vi "op-selector.vi"(6 "Channel":T1={"Operation"=0, "Num. Steps"=0, "Begin"=0.0, "Step Size"=0.0, "Input - A"=0, "Input - B"=0, "Output - LO"=0.0, "Output - HI"=0.0, "Reset"=FALSE, "Analog Output"=0, "Trigger Input"=0, "Initialize To"=0, "Digital Inputs"=[0, 0, 0, 0, 0], "Output Values"=[0.0, 0.0, 0.0, 0.0, 0.0], "Num. Inputs"=4} {"Digital Inputs" items=["DIO0", "DIO1", "DIO2", "DIO3", "DIO4", "DIO5", "DIO6", "DIO7", "DIO8", "DIO9", "DIO10", "DIO11", "DIO12", "DIO13", "DIO14", "DIO15", "DIO16", "DIO17", "DIO18", "DIO19", "DIO20", "DIO21", "DIO22", "DIO23", "DIO24", "DIO25", "DIO26", "DIO27", "DIO28", "DIO29", "DIO30", "DIO31"]; "Initialize To" items=["Zero", "Begin Value"]; "Trigger Input" items=["DIO0", "DIO1", "DIO2", "DIO3", "DIO4", "DIO5", "DIO6", "DIO7", "DIO8", "DIO9", "DIO10", "DIO11", "DIO12", "DIO13", "DIO14", "DIO15", "DIO16", "DIO17", "DIO18", "DIO19", "DIO20", "DIO21", "DIO22", "DIO23", "DIO24", "DIO25", "DIO26", "DIO27", "DIO28", "DIO29", "DIO30", "DIO31"]; "Analog Output" items=["AO\\00", "AO\\01", "AO\\02", "AO\\03", "AO\\04", "AO\\05", "AO\\06", "AO\\07", "AO\\08", "AO\\09", "AO\\10", "AO\\11", "AO\\12", "AO\\13", "AO\\14", "AO\\15"]; "Input - B" items=["DIO0", "DIO1", "DIO2", "DIO3", "DIO4", "DIO5", "DIO6", "DIO7", "DIO8", "DIO9", "DIO10", "DIO11", "DIO12", "DIO13", "DIO14", "DIO15", "DIO16", "DIO17", "DIO18", "DIO19", "DIO20", "DIO21", "DIO22", "DIO23", "DIO24", "DIO25", "DIO26", "DIO27", "DIO28", "DIO29", "DIO30", "DIO31"]; "Input - A" items=["DIO0", "DIO1", "DIO2", "DIO3", "DIO4", "DIO5", "DIO6", "DIO7", "DIO8", "DIO9", "DIO10", "DIO11", "DIO12", "DIO13", "DIO14", "DIO15", "DIO16", "DIO17", "DIO18", "DIO19", "DIO20", "DIO21", "DIO22", "DIO23", "DIO24", "DIO25", "DIO26", "DIO27", "DIO28", "DIO29", "DIO30", "DIO31"]; "Operation" items=["OFF", "SWITCH", "AND GATE", "OR GATE", "ITERATION", "CUSTOM - 461nm Freq."]}, 8 "Prev DIO State":bool[](array[boolean])=[FALSE, FALSE, FALSE, FALSE, FALSE, FALSE, FALSE, FALSE, FALSE, FALSE, FALSE, FALSE, FALSE, FALSE, FALSE, FALSE, FALSE, FALSE, FALSE, FALSE, FALSE, FALSE, FALSE, FALSE, FALSE, FALSE, FALSE, FALSE, FALSE, FALSE, FALSE, FALSE], 9 "Prev AO Values":fxp<+/-,20,5>[](array[numeric])=[0.0, 0.0, 0.0, 0.0, 0.0, 0.0, 0.0, 0.0, 0.0, 0.0, 0.0, 0.0, 0.0, 0.0, 0.0, 0.0], 10 "Iter Counter In":u16[](array[numeric])=[0, 0, 0, 0, 0, 0, 0, 0, 0, 0, 0, 0, 0, 0, 0, 0], 11 "Digital Input Value Array":bool[](array[boolean])=[FALSE, FALSE, FALSE, FALSE, FALSE, FALSE, FALSE, FALSE, FALSE, FALSE, FALSE, FALSE, FALSE, FALSE, FALSE, FALSE, FALSE, FALSE, FALSE, FALSE, FALSE, FALSE, FALSE, FALSE, FALSE, FALSE, FALSE, FALSE, FALSE, FALSE, FALSE, FALSE]) -> (0 "Current DIO State":bool[](array[boolean]), 1 "New AO Values":fxp<+/-,20,5>[](array[numeric]), 2 "Iter Counter Out":u16[](array[numeric]))   [LabVIEW 2016]
uses:
  fpga_array_element.ctl
panel:
  # "IO values for iteration operation"
  # "Boolean Operation Controls"
  # "Iteration Operation Controls"
  # "Custom Operation Controls"
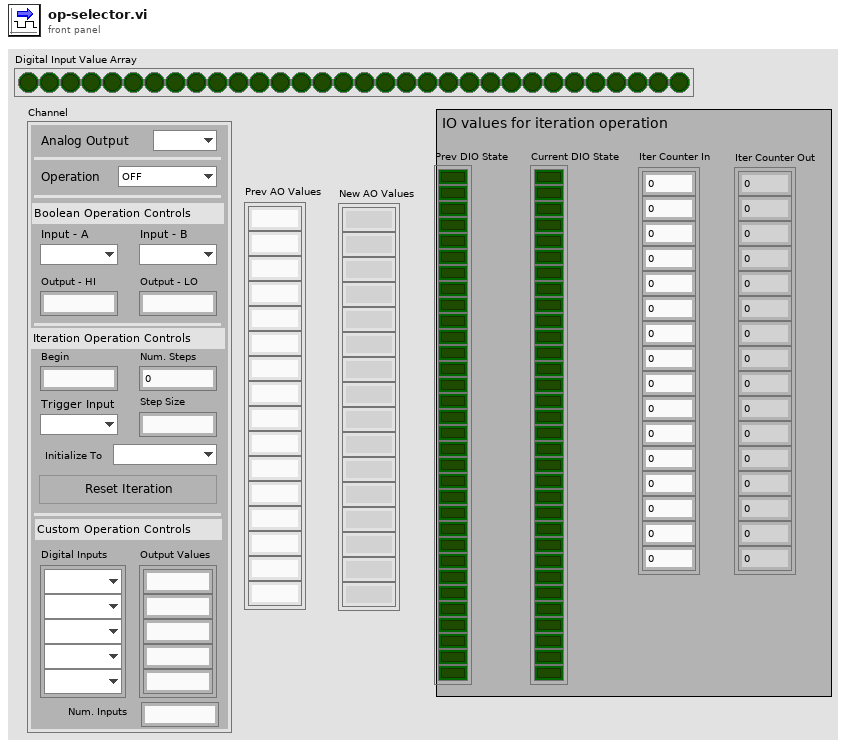
[diagram p1: front panel]
types:
  T1 = typedef "fpga_array_element.ctl" = cluster{"Operation":i16, "Num. Steps":u16, "Begin":fxp<+/-,20,5>, "Step Size":fxp<+/-,20,5>, "Input - A":i32, "Input - B":i32, "Output - LO":fxp<+/-,20,5>, "Output - HI":fxp<+/-,20,5>, "Reset":bool, "Analog Output":i32, "Trigger Input":i32, "Initialize To":i16, "Digital Inputs":i32[], "Output Values":fxp<+/-,20,5>[], "Num. Inputs":u16}
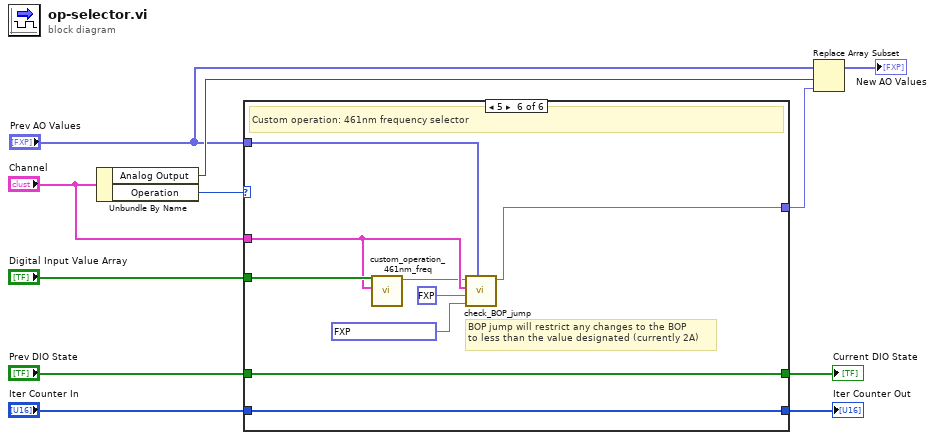
[diagram p0: block diagram]
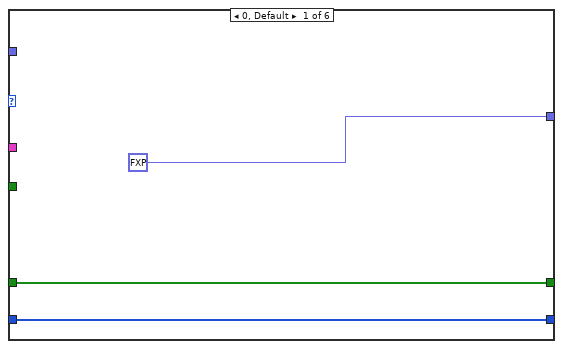
[diagram p2: hidden frame]
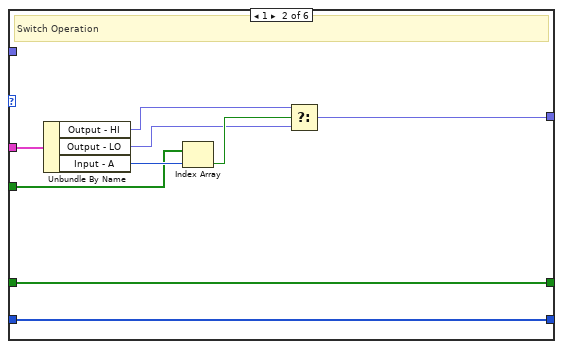
[diagram p3: hidden frame]
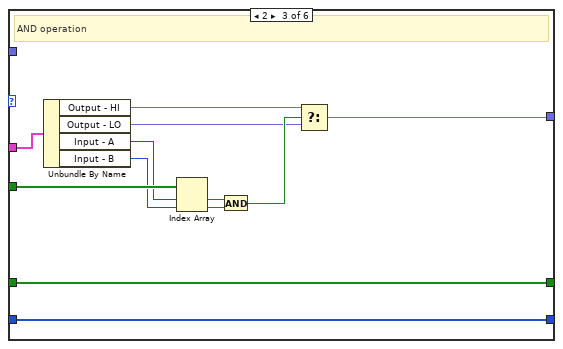
[diagram p4: hidden frame]
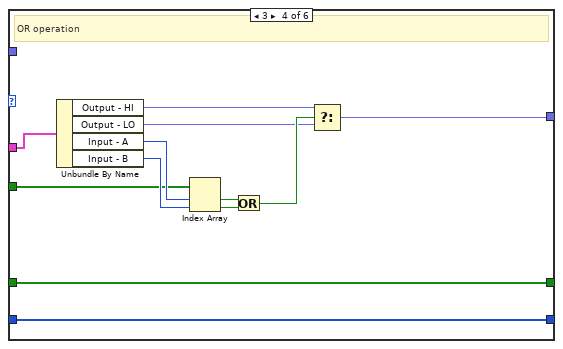
[diagram p5: hidden frame]
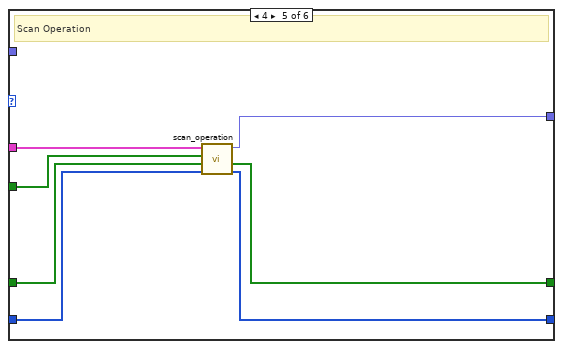
[diagram p6: hidden frame]
diagram:
  n1 = Unbundle By Name("Channel") -> ("Analog Output"=w3:i32, "Operation"=w10:i16)
  n2 = case shown="5" w10 {
    tunnel: [fxp<+,20,5> 0.0 w18 w29 w38 w48 w55] -> w4
    tunnel: "Channel" -> [_ w23 w35 w39 w54 w59]
    tunnel: [w13 w16 w24 w36 w49 w62] -> w6
    tunnel: [w12 w15 w25 w37 w50 w61] -> w5
    tunnel: "Digital Input Value Array" -> [_ w17 w28 w40 w53 w63]
    tunnel: "Prev DIO State" -> [w13 w16 w24 w36 w52 w62]
    tunnel: "Iter Counter In" -> [w12 w15 w25 w37 w51 w61]
    tunnel: "Prev AO Values" -> [_ _ _ _ _ w60]
    frame 0, Default {
    }
    frame 1 {
      # "Switch Operation"
      n3 = Unbundle By Name(w23) -> ("Output - HI"=w19:fxp<+/-,20,5>, "Output - LO"=w20:fxp<+/-,20,5>, "Input - A"=w22:i32)
      n4 = Index Array(array=w17, index=w22) -> (element=w21:bool)
      n5 = Select(t=w19, s=w21, f=w20) -> (s? t:f=w18:fxp<+/-,20,5>)
    }
    frame 2 {
      # "AND operation"
      n6 = Unbundle By Name(w35) -> ("Output - HI"=w31:fxp<+/-,20,5>, "Output - LO"=w30:fxp<+/-,20,5>, "Input - A"=w26:i32, "Input - B"=w27:i32)
      n7 = Index Array(array=w28, index #1=w26, index #2=w27) -> (element #1=w34:bool, element #2=w33:bool)
      n8 = And(x=w34, y=w33) -> (x .and. y?=w32:bool)
      n9 = Select(t=w31, s=w32, f=w30) -> (s? t:f=w29:fxp<+/-,20,5>)
    }
    frame 3 {
      # "OR operation"
      n10 = Unbundle By Name(w39) -> ("Output - HI"=w44:fxp<+/-,20,5>, "Output - LO"=w43:fxp<+/-,20,5>, "Input - A"=w41:i32, "Input - B"=w42:i32)
      n11 = Index Array(array=w40, index #1=w41, index #2=w42) -> (element #1=w47:bool, element #2=w46:bool)
      n12 = Or(x=w47, y=w46) -> (x .or. y?=w45:bool)
      n13 = Select(t=w44, s=w45, f=w43) -> (s? t:f=w38:fxp<+/-,20,5>)
    }
    frame 4 {
      # "Scan Operation"
      n14 = call "scan_operation.vi"("Iter Counter In"=w51, "Prev DIO State"=w52, "Digital Input Value Array"=w53, "Channel"=w54) -> ("Iter Counter Out"=w50:u16[], "Current DIO State"=w49:bool[], "AO out"=w48:fxp<+/-,20,5>)  [unwired: 1 in]
    }
    frame 5 {
      # "BOP jump will restrict any changes to the BOP\nto less than the value designated (currently 2A)"
      # "Custom operation: 461nm frequency selector"
      n15 = call "custom_operation_461nm_freq.vi"("Channel"=w59, "Digital Input Value Array"=w63) -> ("AO Out"=w56:fxp<+/-,20,5>)  [unwired: 9 in]
      n16 = call "check_BOP_jump.vi"("Prev AO Values"=w60, "Increment Amount"=fxp<+/-,20,5> 0.001007080078125, "BOP jump limit"=fxp<+/-,20,5> 1.0, "Channel"=w59, "AO to Check"=w56) -> ("AO Out"=w55:fxp<+/-,20,5>)  [unwired: 6 in]
    }
  }
  "Current DIO State" <- w6
  "Iter Counter Out" <- w5
  n17 = Replace Array Subset(array="Prev AO Values", new element=w4, index=w3) -> (→"New AO Values":fxp<+/-,20,5>[])
